vi "State_Machine.vi"(8 "error in (no error)":errorcluster caption="entrée d'erreur (pas d'erreur)", 11 "Generate_SN en entrée":refnum<class "Generate_SN.lvclass">) -> (0 "error out":errorcluster caption="sortie d'erreur", 2 "Json_String":string, 3 "Generate_SN en sortie":refnum<class "Generate_SN.lvclass">)   [LabVIEW 2020, in "Library Test.lvlib" / "Generate_SN.lvclass"]
uses:
  Generate_SN.lvclass
  C:/Users/ngarcin/OneDrive - Altyor/Standard TB/Suite TB45/Class/Test/Test (Default)/Test (Default).lvclass
  Creation_SN/Creation_SN Database (Default)/Creation_SN Database (Default).lvclass
  C:/Users/ngarcin/OneDrive - Altyor/Standard TB/Suite TB45/Class/Creation_SN/Creation_SN (Default)/Creation_SN (Virtual).lvclass
  Commun VI/TypeDef/Variable Printable.ctl
  Commun VI/TypeDef/Liste Error.ctl
  Creation_SN/Creation_SN_P2265/Creation_SN_P2265.lvclass
  C:/Users/ngarcin/OneDrive - Altyor/Standard TB/Suite TB45/Class/Creation_SN/Creation_SN Database (Default)/Creation_SN Database (Default).lvclass
  Creation_SN/Creation_SN_P2222/Creation_SN_P2222.lvclass
  Creation_SN/Creation_SN_Nodon/Creation_SN_Nodon.lvclass
  JSON API/JSON Value/Set from JSON string.vi
  Instrument/Instrument (Default)/Class Instrument (Default).lvclass
  JSON API/JSON Value/JSON Value.lvclass
  JSON API/Variant JSON/Variant JSON.lvlib
  JSON API/Get Polymorphic/JSON GetSet.lvlib
  Commun VI/Library Commun.lvlib
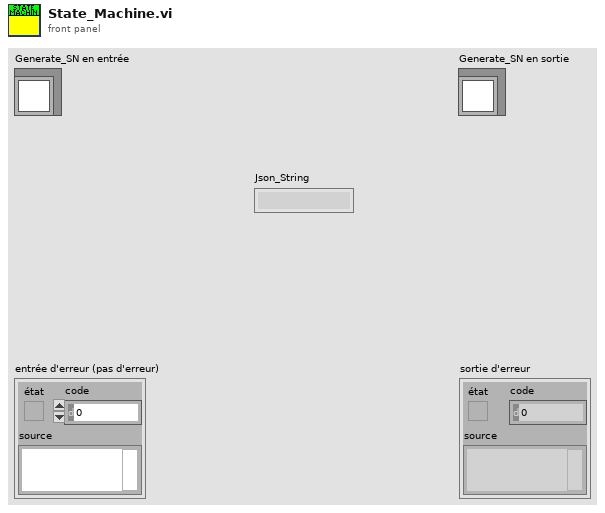
[diagram p1: front panel]
types:
  T1 = typedef "Variable Printable.ctl" = string
  T2 = enum16{"Get Variable", "Get All Variables", "Set Variable", "Delete Variable", "Delete All Variable"}
  T3 = typedef "Library Commun.lvlib/Liste Error.ctl" = enum16{"Firebase Driver - Get Document", "Firebase Driver - Get Document With Where", "Firebase Driver - Delete Document", "Firebase Driver - Set Document", "Firebase Driver - Update Document", "Firebase Altyor - Search Document Bench", "Firebase Altyor - Class Not in Firebase", "Spectrum_Analyser - Timeout", "Relay Board - Qty Relay", "DIO - Pb Funtion", "Power_Supply - Peripherical not find", "Mutimeter - Peripherical not find", "Instrument - Function Not Used", "Instrument - Instrument name not specified", "Instrument - Allready Initialised", "Instrument - TimeOut", "Instrument - the instrument must be Initialise before", "Instrument - Frame Not received", "Instrument - Frame Nok", "Test - Initialise the File_for_Save", "Test - Timeout", "Test - Cmd Error", "FGV - Variable ", "BDD FireBase - Define Class", "SN - Class Not Define"}
  T4 = cluster{"Protocol":string, "Product Number":string}
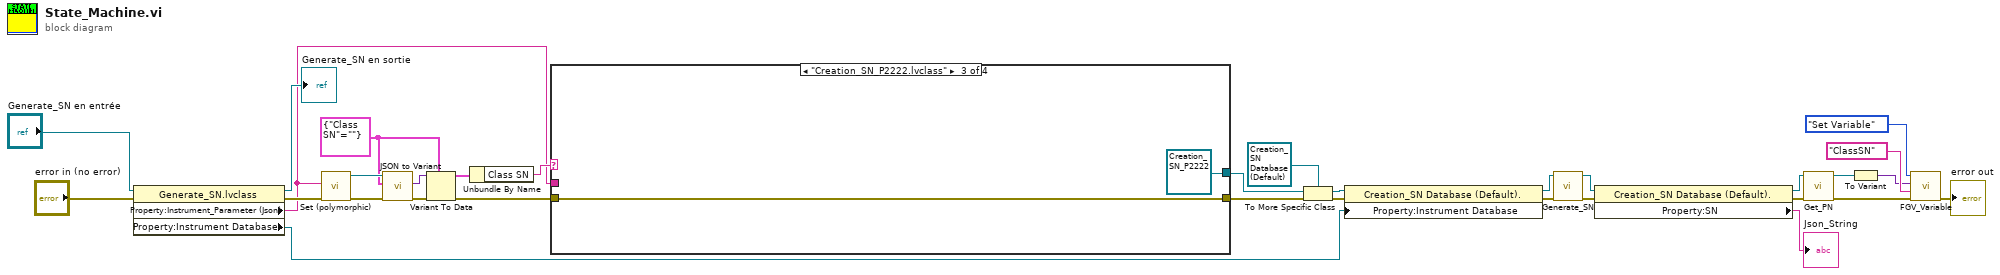
[diagram p0: block diagram]
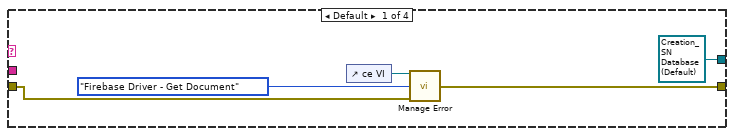
[diagram p2: hidden frame]
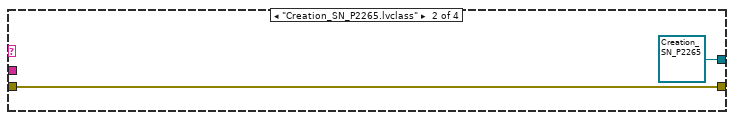
[diagram p3: hidden frame]
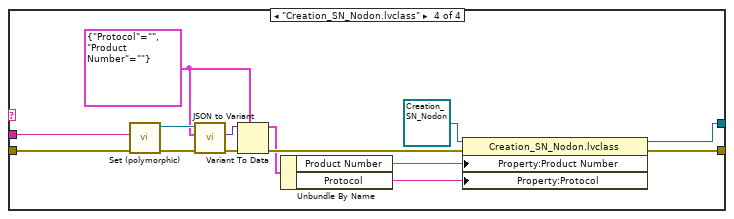
[diagram p4: hidden frame]
diagram:
  w3 = cluster{"Class SN":string} {"Class SN"=""}
  n1 = property class="Generate_SN.lvclass"(reference="Generate_SN en entrée", error in="error in (no error)") -> (reference out=→"Generate_SN en sortie":refnum<class "Generate_SN.lvclass">, error out=w18:errorcluster, "Property:Instrument_Parameter (Json)"=w1:string, "Property:Instrument Database"=w29:refnum<class "Class Instrument (Default).lvclass">)
  n2 = call-poly "Set (polymorphic).vi"("error in (no error)"=w18, "JSON stream"=w1) -> ("error out"=w20:errorcluster, "JSON Value out"=w22:refnum<class "JSON Value.lvclass">)  [unwired: 7 in, 1 out]
  n3 = call "JSON to Variant.vi"("error in (no error)"=w20, "Variant (Data Type)"=w3, "JSON Value"=w22) -> ("error out"=w21:errorcluster, "Variant out"=w19:variant)  [unwired: 7 in]
  n4 = Variant To Data(error in=w21, type=w3, Variant=w19) -> (data=w17:cluster{"Class SN":string}, error out=w15:errorcluster)
  n5 = Unbundle By Name(w17) -> ("Class SN"=w2:string)
  n6 = case shown="\"Creation_SN_P2222.lvclass\"" w2 {
    tunnel: [refnum<class "Creation_SN Database (Default).lvclass"> refnum ("Library Creation_SN.lvlib:Creation_SN Database (Default).lvclass") refnum<class "Creation_SN_P2265.lvclass"> refnum ("Library Creation_SN.lvlib:Creation_SN_P2265.lvclass") refnum<class "Creation_SN_P2222.lvclass"> refnum ("Library Instrument & Equipement.lvlib:Library Creation_SN.lvlib:Creation_SN_P2222.lvclass") w54] -> w25
    tunnel: w15 -> [w35 w38 w41 w48]
    tunnel: [w34 w38 w41 w53] -> w14
    tunnel: w1 -> [_ _ _ w46]
    frame Default {
      n7 = control-ref of="ce VI"() -> (w33:refnum<vi>)
      n8 = call "Manage Error.vi"("VI in Error"=w33, "Code Erreur"=Liste_Error."Firebase Driver - Get Document", "error in (no error)"=w35) -> ("error out"=w34:errorcluster)  [unwired: 12 in]
    }
    frame "Creation_SN_P2265.lvclass" {
    }
    frame "Creation_SN_P2222.lvclass" {
    }
    frame "Creation_SN_Nodon.lvclass" {
      w42 = T4 {"Protocol"="", "Product Number"=""}
      n9 = call-poly "Set (polymorphic).vi"("error in (no error)"=w48, "JSON stream"=w46) -> ("error out"=w51:errorcluster, "JSON Value out"=w49:refnum<class "JSON Value.lvclass">)  [unwired: 7 in, 1 out]
      n10 = call "JSON to Variant.vi"("error in (no error)"=w51, "Variant (Data Type)"=w42, "JSON Value"=w49) -> ("error out"=w50:errorcluster, "Variant out"=w52:variant)  [unwired: 7 in]
      n11 = Variant To Data(error in=w50, type=w42, Variant=w52) -> (data=w45:T4, error out=w47:errorcluster)
      n12 = Unbundle By Name(w45) -> ("Product Number"=w43:string, "Protocol"=w44:string)
      n13 = property class="Creation_SN_Nodon.lvclass"(reference=refnum<class "Creation_SN_Nodon.lvclass"> refnum ("Library Creation_SN.lvlib:Creation_SN_Nodon.lvclass"), error in=w47, "Property:Product Number"=w43, "Property:Protocol"=w44) -> (reference out=w54:refnum<class "Creation_SN_Nodon.lvclass">, error out=w53:errorcluster)
    }
  }
  n14 = To More Specific Class(target class=refnum<class "Creation_SN Database (Default).lvclass"> refnum ("Library Creation_SN.lvlib:Creation_SN Database (Default).lvclass"), reference=w25, error in=w14) -> (specific class reference=w24:refnum<class "Creation_SN Database (Default).lvclass">, error out=w16:errorcluster)
  n15 = property class="Creation_SN Database (Default)."(reference=w24, error in=w16, "Property:Instrument Database"=w29) -> (reference out=w31:refnum<class "Creation_SN Database (Default).lvclass">, error out=w23:errorcluster)
  n16 = call-dynamic "Generate_SN.vi"("error in (no error)"=w23, "Class Creation_SN (Default) en entrée"=w31) -> ("error out"=w5:errorcluster, "Class Creation_SN (Default) en sortie"=w30:refnum<class "Creation_SN Database (Default).lvclass">)  [unwired: 8 in]
  n17 = property class="Creation_SN Database (Default)."(reference=w30, error in=w5) -> (reference out=w7:refnum<class "Creation_SN Database (Default).lvclass">, error out=w4:errorcluster, "Property:SN"=→"Json_String":string)
  n18 = call-dynamic "Get_PN.vi"("error in (no error)"=w4, "Class Creation_SN (Default) en entrée"=w7) -> ("error out"=w13:errorcluster, "Class Creation_SN (Default) en sortie"=w9:refnum<class "Creation_SN Database (Default).lvclass">)  [unwired: 8 in]
  n19 = To Variant(anything=w9) -> (Variant=w8:variant)
  n20 = call "FGV_Variable.vi"("error in (no error)"=w13, "Variable"=T1 "ClassSN", "Data In"=w8, "Function"=T2."Set Variable") -> ("error out"=→"error out":errorcluster)  [unwired: 5 in, 2 out]
